vi "HV Open Another App.vi"(11 "Vi Name":string="/HV Append V_Settings.vi") -> (3 "standard output":string)   [LabVIEW 2018, in "HV QMH.lvlib"]
doc: "This example allows to choose a VI to open and run programmatically, then closes the front panel after completion."
uses:
  HV QMH.lvlib
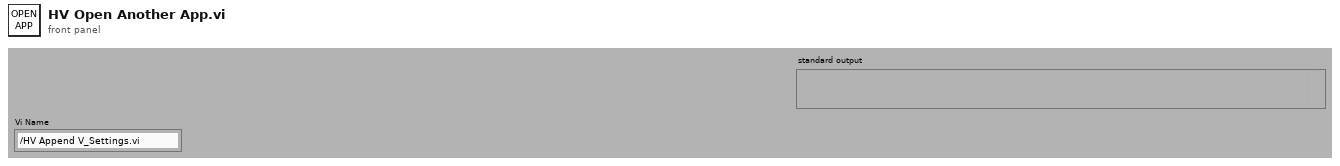
[diagram p1: front panel]
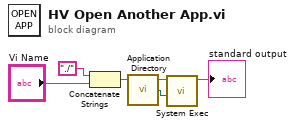
[diagram p0: block diagram]
diagram:
  n1 = Concatenate Strings("./" ("string"), "Vi Name") -> (w2:string)
  n2 = call <vilib>:"Application Directory.vi"() -> ("Application Directory"=w5:path)
  n3 = call <vilib>:"System Exec.vi"("working directory"=w5, "command line"=w2) -> ("standard output"=→"standard output":string)  [unwired: 6 in, 3 out]
